vi "Rename Item.vi"(8 "error in (no error)":errorcluster, 9 "New Item Name":string, 10 "Item Name":string, 11 "Module Name":string) -> (0 "error out":errorcluster)   [LabVIEW 2020, in "Grouped Interface.lvlib"]
uses:
  Grouped Interface.lvlib
  b0072e6c-90f1-4b20-bb3c-1cbdcd159640.vi
  <userlib>/_NEVSTOP/Communicable State Machine(CSM)/addons/API-String-Arugments-Support/_Support/Data To API String Arguments.vi
  <userlib>/_NEVSTOP/Communicable State Machine(CSM)/Communicable State Machine.lvlib
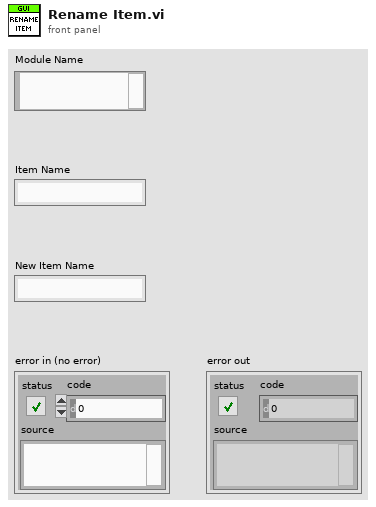
[diagram p1: front panel]
types:
  T1 = cluster{"Item Name":string, "New Item Name":string}
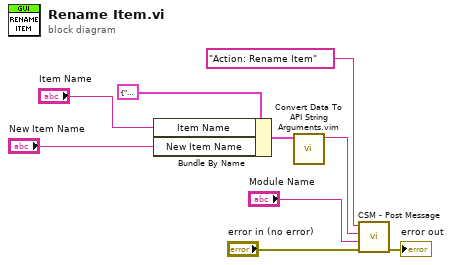
[diagram p0: block diagram]
diagram:
  n1 = Bundle By Name(cluster=T1 {"Item Name"="", "New Item Name"=""}, "Item Name"="Item Name", "New Item Name"="New Item Name") -> (w4:T1)
  n2 = call "Convert Data To API String Arguments.vim"("Data"=w4) -> ("API String"=w3:string)  [unwired: 7 in, 1 out]
  n3 = call <userlib>:"CSM - Post Message.vi"("Error In (No Error)"="error in (no error)", "Target Module"="Module Name", "Arguments (\"\")"=w3, "State"="Action: Rename Item") -> ("error out"=→"error out":errorcluster)  [unwired: 7 in]
